vi "ElevatedPass.vi"(7 "PassState":T1=enum."Pass", 8 "error in (no error)":errorcluster) -> (0 "error out":errorcluster)   [LabVIEW 2015]
doc: "Wrapper for elevated pass. It has the following actions:\n-Pass: sets the clapper to out, the roller motor to reverse, and then sets the roller pneumatic to out.\n-Stop: sets the roller pneumatic to middle, the clapper to in, and the roller motor to off."
uses:
  PassState.ctl
  RollerAction.ctl
  DoubleSolenoidAction.ctl
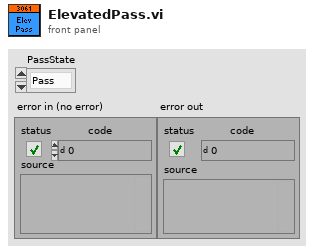
[diagram p1: front panel]
types:
  T1 = typedef "PassState.ctl" = enum16{"Stop", "Pass"}
  T2 = typedef "DoubleSolenoidAction.ctl" = enum16{"Init", "Middle", "In", "Out"}
  T3 = typedef "RollerAction.ctl" = enum16{"Init", "Off", "Forward", "Reverse"}
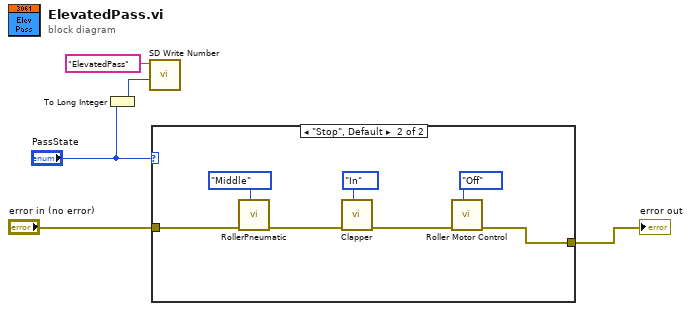
[diagram p0: block diagram]
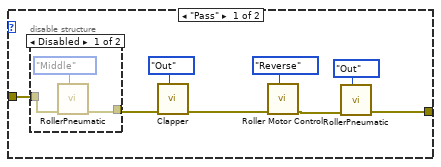
[diagram p2: hidden frame]
diagram:
  n1 = To Long Integer(number="PassState") -> (32bit integer=w2:i32)
  n2 = call <vilib>:"SD Write Number.vi"("Numeric"=w2, "Name"="ElevatedPass") -> ()  [unwired: 8 in, 2 out]
  n3 = case shown="\"Stop\", Default" "PassState" {
    tunnel: "error in (no error)" -> [w8 w18]
    tunnel: [w7 w17] -> w4
    frame "Pass" {
      n4 = disable-structure shown="Disabled" {
        disable-tunnel: [w15 _] -> w10
        disable-tunnel: w8 -> [w14 _]
        frame Disabled {
          n5 = call "RollerPneumatic.vi"("State"=DoubleSolenoidAction."Middle", "Error in"=w14) -> ("Error out"=w15:errorcluster)  [unwired: 9 in]
        }
        frame Enabled {
        }
      }
      n6 = call "Clapper.vi"("State"=DoubleSolenoidAction."Out", "Error in"=w10) -> ("Error out"=w11:errorcluster)  [unwired: 9 in]
      n7 = call "Roller Motor Control.vi"("Action"=RollerAction."Reverse", "Error in"=w11) -> ("Error out"=w9:errorcluster)  [unwired: 9 in]
      n8 = call "RollerPneumatic.vi"("State"=DoubleSolenoidAction."Out", "Error in"=w9) -> ("Error out"=w7:errorcluster)  [unwired: 9 in]
    }
    frame "Stop", Default {
      n9 = call "RollerPneumatic.vi"("State"=DoubleSolenoidAction."Middle", "Error in"=w18) -> ("Error out"=w19:errorcluster)  [unwired: 9 in]
      n10 = call "Clapper.vi"("State"=DoubleSolenoidAction."In", "Error in"=w19) -> ("Error out"=w20:errorcluster)  [unwired: 9 in]
      n11 = call "Roller Motor Control.vi"("Action"=RollerAction."Off", "Error in"=w20) -> ("Error out"=w17:errorcluster)  [unwired: 9 in]
    }
  }
  "error out" <- w4
